vi "Pic Overlay bp Point.vi"(8 "error in (no error)":errorcluster, 10 "Picture in":picture, 11 "LF2R IDE in":refnum<class "Main Panel.lvclass">) -> (0 "error out":errorcluster, 2 "Picture out":picture, 3 "LF2R IDE out":refnum<class "Main Panel.lvclass">)   [LabVIEW 2018, in "Main Panel.lvlib" / "Main Panel.lvclass"]
uses:
  Main Panel.lvclass
  Main Panel.lvclass/Main Panel.ctl
  Picture Process/Picture Process.lvclass
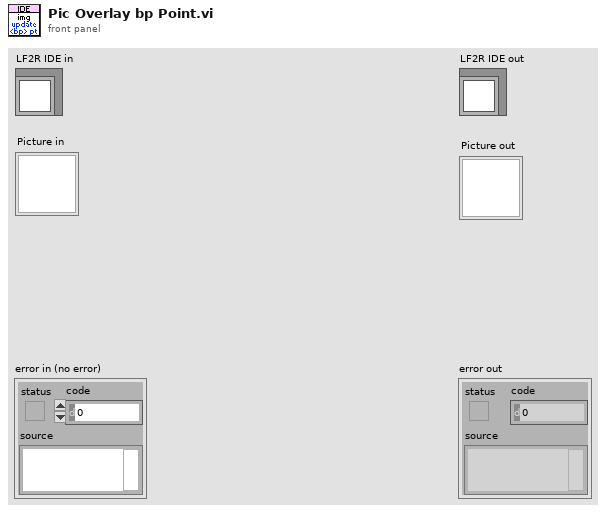
[diagram p1: front panel]
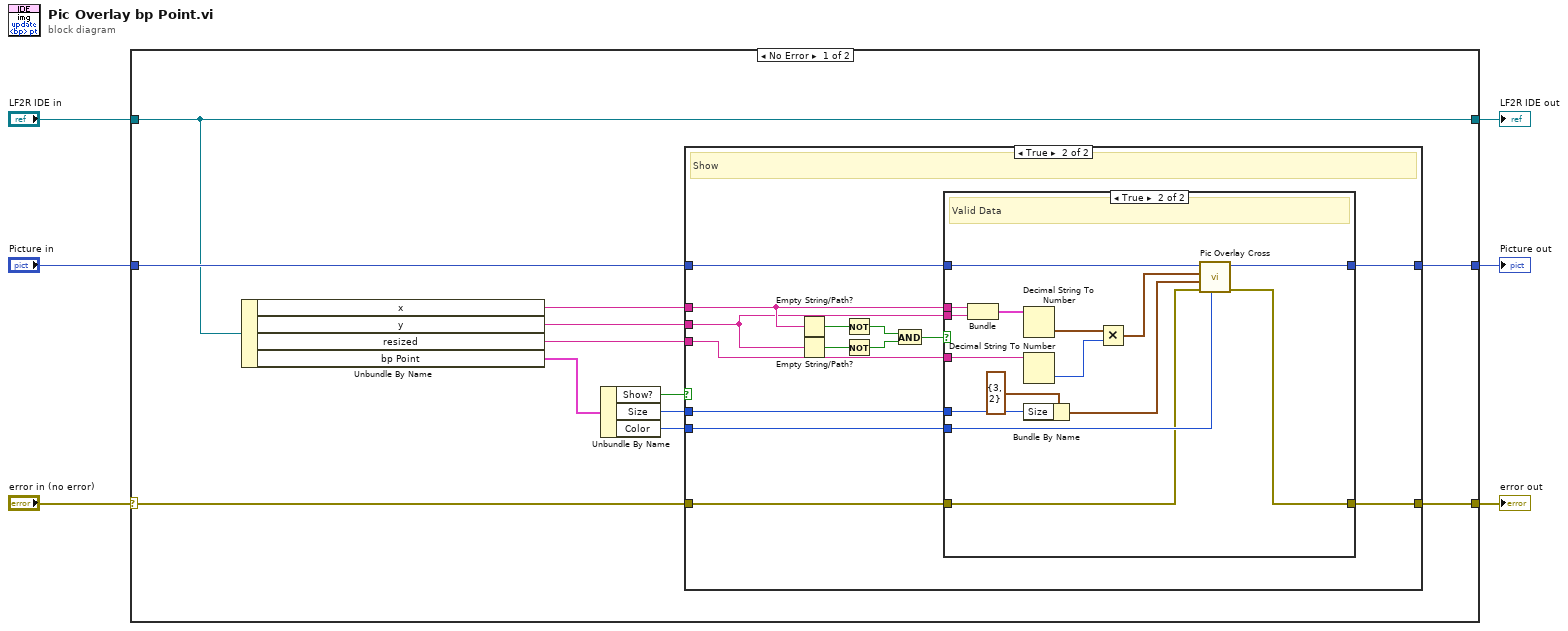
[diagram p0: block diagram]
diagram:
  n1 = case shown="No Error" "error in (no error)" {
    selector: "error in (no error)" -> [w10 w54]
    tunnel: [w8 w54] -> w5
    tunnel: [w9 w53] -> w3
    tunnel: "LF2R IDE in" -> [w9 w53]
    tunnel: "Picture in" -> [w11 w52]
    tunnel: [w7 w52] -> w1
    frame No Error {
      n2 = Unbundle By Name(w9) -> ("x"=w17:string, "y"=w16:string, "resized"=w18:string, "bp Point"=w15:cluster{"Size":i32, "Color":u32, "Show?":bool})
      n3 = Unbundle By Name(w15) -> ("Show?"=w14:bool, "Size"=w13:i32, "Color"=w12:u32)
      n4 = case shown="True" w14 {
        tunnel: w18 -> [_ w34]
        tunnel: w17 -> [_ w33]
        tunnel: w16 -> [_ w32]
        tunnel: w13 -> [_ w26]
        tunnel: w12 -> [_ w25]
        tunnel: w11 -> [w20 w24]
        tunnel: [w20 w23] -> w7
        tunnel: w10 -> [w19 w22]
        tunnel: [w19 w21] -> w8
        frame False {
        }
        frame True {
          # "Show"
          n5 = Empty String/Path?(string/path=w33) -> (empty?=w31:bool)
          n6 = Empty String/Path?(string/path=w32) -> (empty?=w30:bool)
          n7 = Not(x=w31) -> (.not. x?=w29:bool)
          n8 = Not(x=w30) -> (.not. x?=w28:bool)
          n9 = And(x=w29, y=w28) -> (x .and. y?=w27:bool)
          n10 = case shown="True" w27 {
            tunnel: w34 -> [_ w51]
            tunnel: w33 -> [_ w48]
            tunnel: w32 -> [_ w47]
            tunnel: w26 -> [_ w43]
            tunnel: w25 -> [_ w41]
            tunnel: w24 -> [w35 w40]
            tunnel: [w35 w39] -> w23
            tunnel: w22 -> [w36 w38]
            tunnel: [w36 w37] -> w21
            frame False {
              # "Invalid"
            }
            frame True {
              # "Valid Data"
              n11 = Bundle("x"=w48, "y"=w47) -> (w46:cluster{"x":string, "y":string})  [unwired: 1 in]
              n12 = Decimal String To Number(string=w46) -> (number=w50:cluster{"x":i32, "y":i32})  [unwired: 2 in, 1 out]
              n13 = Decimal String To Number(string=w51) -> (number=w49:i32)  [unwired: 2 in, 1 out]
              n14 = Bundle By Name(cluster=cluster{"Size":i32, "Width":u16} {"Size"=3, "Width"=2} ("Line"), "Size"=w43) -> (w42:cluster{"Size":i32, "Width":u16})
              n15 = Multiply(x=w50, y=w49) -> (x*y=w45:cluster{"x":i32, "y":i32})
              n16 = call "Pic Overlay Cross.vi"("Color"=w41, "error in (no error)"=w38, "Line"=w42, "Position"=w45, "Picture in"=w40) -> ("error out"=w37:errorcluster, "Picture out"=w39:picture)  [unwired: 5 in]
            }
          }
        }
      }
    }
    frame Error {
    }
  }
  "error out" <- w5
  "LF2R IDE out" <- w3
  "Picture out" <- w1
